vi "TestSave_NextStep.vi"(8 "error in":errorcluster, 10 "SaveTestData":T1={"data"=[], "TestData"={"FilesPath"=path "", "Name_Meas"="", "stop"=FALSE, "Command"=enum."End", "Fs"=1000.0, "Test"=FALSE}, "Counter"=0.0}, 11 "Previous Step":T4) -> (0 "error out":errorcluster, 3 "Next Step":T4)   [LabVIEW 2019]
uses:
  TypeDef/#TypeDef_StateAcq.ctl
  TypeDef/#TypeDef_SaveTestData.ctl
  TypeDef/#TypeDef_DataToTest.ctl
  Communication/TypeDef/#TypeDef_Command.ctl
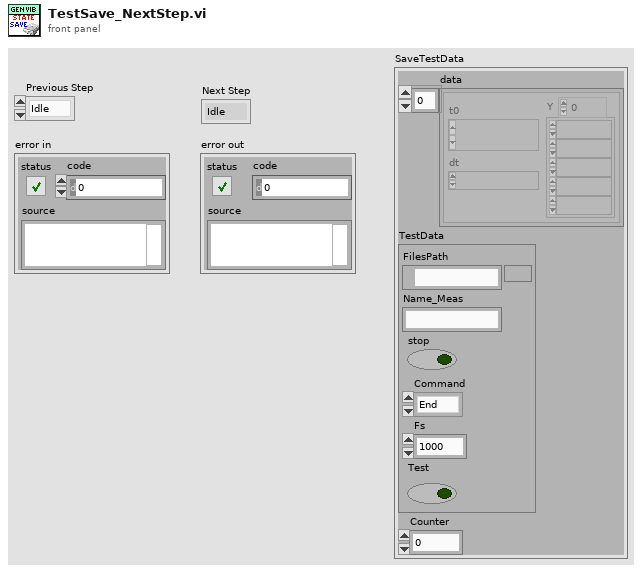
[diagram p1: front panel]
types:
  T1 = typedef "#TypeDef_SaveTestData.ctl" = cluster{"data":waveform(dbl)[], "TestData":T2, "Counter":dbl}
  T2 = typedef "#TypeDef_DataToTest.ctl" = cluster{"FilesPath":path, "Name_Meas":string, "stop":bool, "Command":T3, "Fs":dbl, "Test":bool}
  T3 = typedef "#TypeDef_Command.ctl" = enum16{"Start", "End"}
  T4 = typedef "#TypeDef_StateAcq.ctl" = enum16{"Idle", "Init", "Acq", "End"}
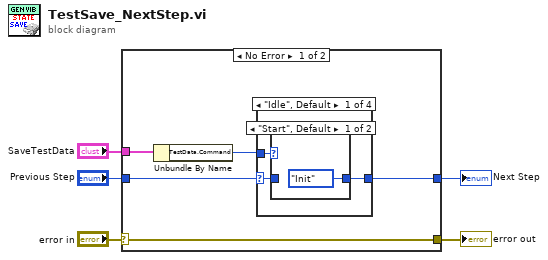
[diagram p0: block diagram]
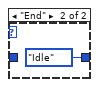
[diagram p2: hidden frame]
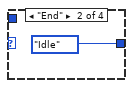
[diagram p3: hidden frame]
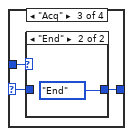
[diagram p4: hidden frame]
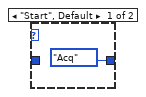
[diagram p5: hidden frame]
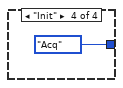
[diagram p6: hidden frame]
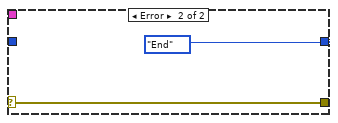
[diagram p7: hidden frame]
diagram:
  n1 = case shown="No Error" "error in" {
    selector: "error in" -> [w10 w24]
    tunnel: [w10 w24] -> w2
    tunnel: [w8 #TypeDef_StateAcq."End"] -> w5
    tunnel: "Previous Step" -> [w9 _]
    tunnel: "SaveTestData" -> [w7 _]
    frame No Error {
      n2 = Unbundle By Name(w7) -> ("TestData.Command"=w6:T3)
      n3 = case shown="\"Idle\", Default" w9 {
        selector: w9 -> [w12 _ w18 _]
        tunnel: w6 -> [w13 _ w17 _]
        tunnel: [w11 #TypeDef_StateAcq."Idle" w19 #TypeDef_StateAcq."Acq"] -> w8
        frame "Idle", Default {
          n4 = case shown="\"Start\", Default" w13 {
            tunnel: [#TypeDef_StateAcq."Init" #TypeDef_StateAcq."Idle"] -> w11
            tunnel: w12 -> [_ _]
            frame "Start", Default {
            }
            frame "End" {
            }
          }
        }
        frame "End" {
        }
        frame "Acq" {
          n5 = case shown="\"End\"" w17 {
            tunnel: [#TypeDef_StateAcq."Acq" #TypeDef_StateAcq."End"] -> w19
            tunnel: w18 -> [_ _]
            frame "Start", Default {
            }
            frame "End" {
            }
          }
        }
        frame "Init" {
        }
      }
    }
    frame Error {
    }
  }
  "error out" <- w2
  "Next Step" <- w5
